vi "presets2 dialog.vi"(11 "Countries in":i32[](array[numeric])) -> (2 "Load?":bool, 3 "Countries out":i32[](array[numeric]))   [LabVIEW 2019]
uses:
  <vilib>/Utility/sysdir.llb/System Directory Type.ctl
  <vilib>/Utility/config.llb/Write Key (I32).vi
  <vilib>/Utility/config.llb/Read Key (I32).vi
  <vilib>/Utility/config.llb/NI_LVConfig.lvlib
panel:
  in  "Delete":bool
  in  "Load":bool
  in  "Save Button":bool
  in  "Cancel Button":bool
  in  "Presets":i32(listbox)
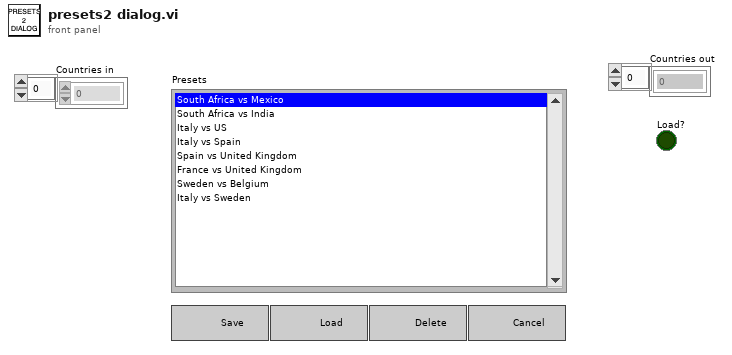
[diagram p1: front panel]
types:
  T1 = typedef "System Directory Type.ctl" = i32
  T2 = typedef "NI_LVConfig.lvlib/Config Data RefNum.ctl" = refnum<k1>
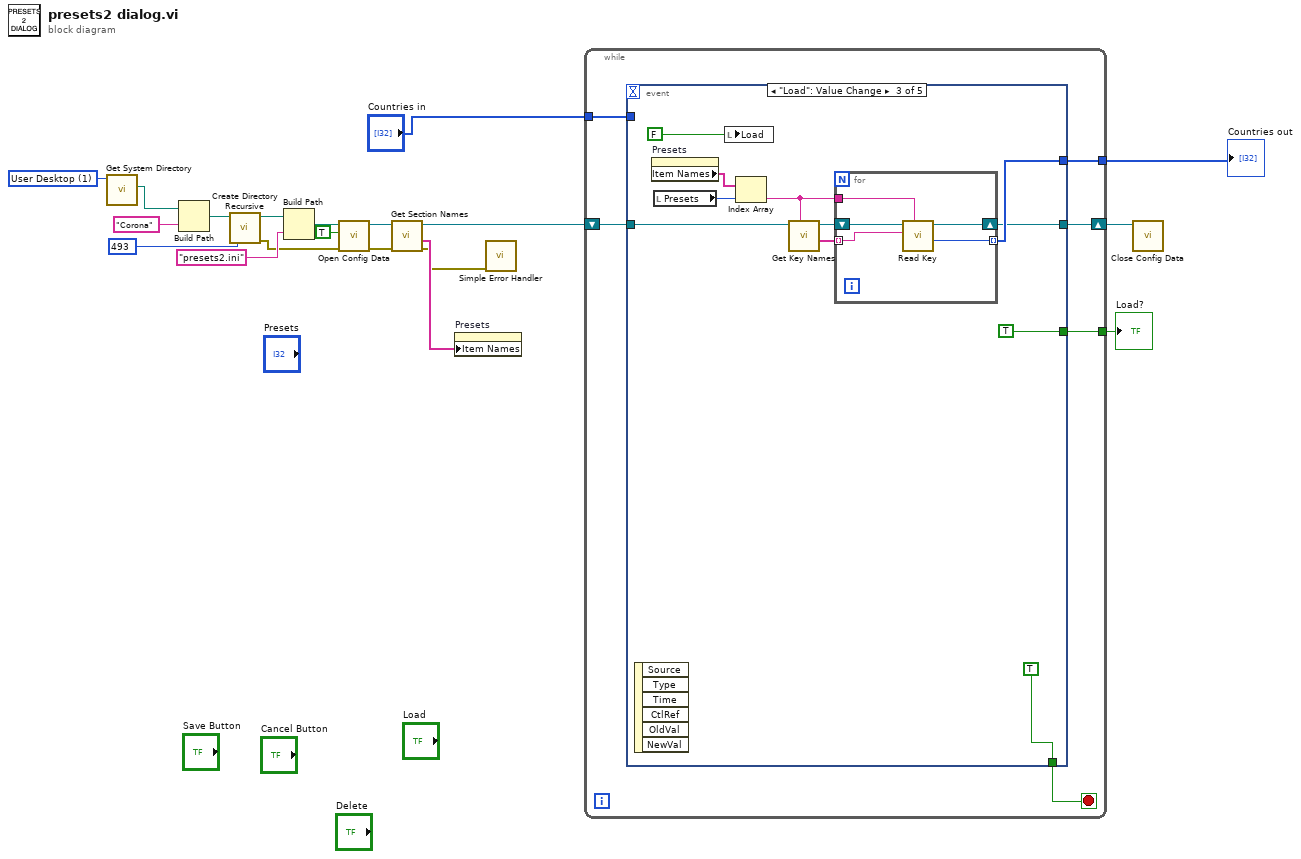
[diagram p0: block diagram]
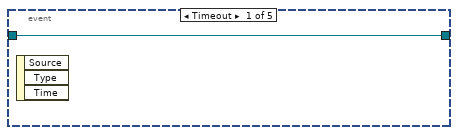
[diagram p2: hidden frame]
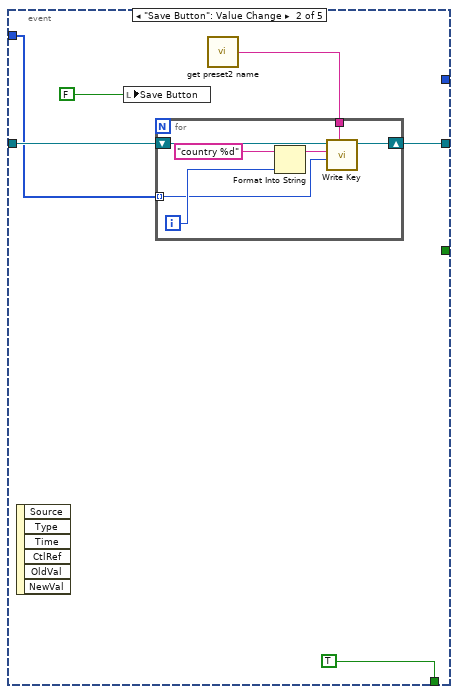
[diagram p3: hidden frame]
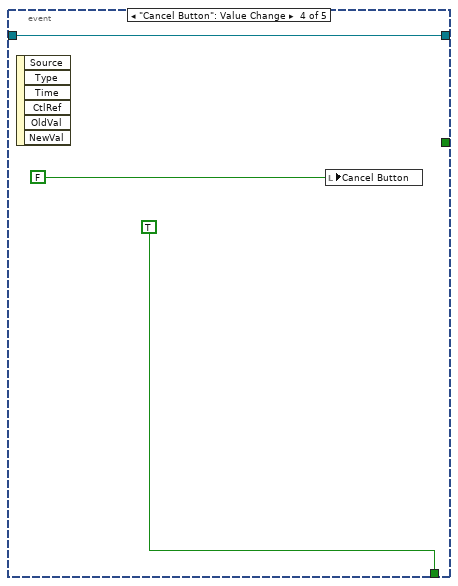
[diagram p4: hidden frame]
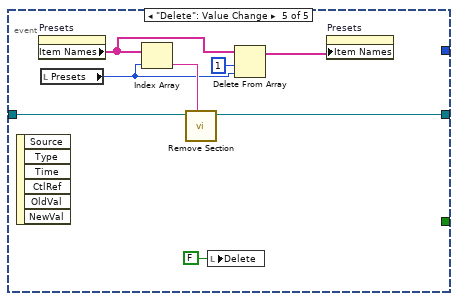
[diagram p5: hidden frame]
diagram:
  w19 = T1 1 items=["User Home"=0, "User Desktop"=1, "User Documents"=2, "User Application Data"=3, "User Preferences"=4, "User Temporary"=5, "Public Documents"=6, "Public Application Data"=7, "Public Preferences"=8, "Public Cache"=13, "System Core Libraries"=9, "System Installed Libraries"=10, "Application Files"=11, "Boot Volume Root"=12] ("system directory type")
  n1 = call <vilib>:"Get System Directory.vi"("system directory type"=w19) -> ("system directory"=w18:path)  [unwired: 10 in]
  n2 = Build Path(base path=w18, name or relative path="Corona") -> (appended path=w7:path)
  n3 = call <vilib>:"Create Directory Recursive.vi"("permissions"=i16 493, "directory"=w7) -> ("error out"=w5:errorcluster, "directory copy"=w6:path)  [unwired: 3 in, 1 out]
  n4 = Build Path(base path=w6, name or relative path="presets2.ini") -> (appended path=w15:path)
  n5 = call <vilib>:"Open Config Data.vi"("error in (no error)"=w5, "create file if necessary (T)"=TRUE, "configuration file path"=w15) -> ("error out"=w9:errorcluster, "refnum"=w13:T2)  [unwired: 6 in, 1 out]
  n6 = call <vilib>:"Get Section Names.vi"("error in (no error)"=w9, "refnum"=w13) -> ("error out"=w8:errorcluster, "section names"=w11:string[], "refnum out"=w12:T2)  [unwired: 7 in]
  n7 = property on="Presets" class="LstBox (strict)"("Item Names"=w11) -> ()  [unwired: 2 in, 2 out]
  n8 = call <vilib>:"Simple Error Handler.vi"("error in (no error)"=w8) -> ()  [unwired: 4 in, 5 out]
  n9 = while {
    shift-right: [w24] -> w10
    shift-left: w12 -> [w25]
    tunnel: "Countries in" -> [w22]
    tunnel: [w21] -> w2
    tunnel: [w20] -> w3
    stop <- w23 stop-if-true
    n10 = event shown="[2] \"Load\": Value Change" {
      selector: _ -> [_ _ _ _ _]
      dyn-events: _ -> [_ _ _ _ _]
      timeout: _ -> [_ _ _ _ _]
      tunnel: w25 -> [w26 w32 w45 w57 w66]
      tunnel: [w26 w27 w41 w57 w64] -> w24
      tunnel: [_ TRUE TRUE TRUE _] -> w23
      tunnel: w22 -> [_ w28 _ _ _]
      tunnel: [_ _ w42 _ _] -> w21
      tunnel: [_ _ TRUE _ _] -> w20
      event Timeout {
        n11 = event-data() -> ()  [unwired: 1 in, 3 out]
      }
      event "Save Button": Value Change {
        n12 = event-data() -> ()  [unwired: 1 in, 6 out]
        n13 = local write "Save Button"(FALSE ("Save Button")) -> ()
        n14 = call "get preset2 name.vi"() -> ("Preset name out"=w29:string)  [unwired: 1 in]
        n15 = for {
          tunnel: w29 -> [w37]
          tunnel: w28 -> [w34] mode=indexing
          shift-right: [w33] -> w27
          shift-left: w32 -> [w39]
          i -> [w35]
          n16 = Format Into String(initial string="country %d" ("key"), w35) -> (resulting string=w36:string)  [unwired: 2 in, 1 out]
          n17 = call-poly <vilib>:"Write Key.vi"("section"=w37, "value"=w34, "key"=w36, "refnum"=w39) -> ("refnum out"=w33:T2)  [unwired: 5 in, 2 out]
        }
      }
      event "Load": Value Change {
        n18 = event-data() -> ()  [unwired: 1 in, 6 out]
        n19 = property on="Presets" class="LstBox (strict)"() -> ("Item Names"=w48:string[])  [unwired: 2 in, 2 out]
        n20 = local read "Presets"() -> (w47:i32)
        n21 = local write "Load"(FALSE ("Save Button")) -> ()
        n22 = Index Array(array=w48, index=w47) -> (element=w40:string)
        n23 = call <vilib>:"Get Key Names.vi"("section"=w40, "refnum"=w45) -> ("key names"=w43:string[], "refnum out"=w44:T2)  [unwired: 6 in, 2 out]
        n24 = for {
          tunnel: w43 -> [w52] mode=indexing
          shift-right: [w54] -> w41
          shift-left: w44 -> [w55]
          tunnel: [w53] -> w42 mode=indexing
          tunnel: w40 -> [w51]
          n25 = call-poly <vilib>:"Read Key.vi"("section"=w51, "key"=w52, "refnum"=w55) -> ("value"=w53:i32, "refnum out"=w54:T2)  [unwired: 5 in, 2 out]
        }
      }
      event "Cancel Button": Value Change {
        n26 = event-data() -> ()  [unwired: 1 in, 6 out]
        n27 = local write "Cancel Button"(FALSE ("Cancel Button")) -> ()
      }
      event "Delete": Value Change {
        n28 = event-data() -> ()  [unwired: 1 in, 6 out]
        n29 = property on="Presets" class="LstBox (strict)"() -> ("Item Names"=w63:string[])  [unwired: 2 in, 2 out]
        n30 = local read "Presets"() -> (w61:i32)
        n31 = Index Array(array=w63, index=w61) -> (element=w65:string)
        n32 = call <vilib>:"Remove Section.vi"("section"=w65, "refnum"=w66) -> ("refnum out"=w64:T2)  [unwired: 7 in, 2 out]
        n33 = local write "Delete"(FALSE ("Delete")) -> ()
        n34 = Delete From Array(array=w63, length=1, index=w61) -> (array with subset deleted=w62:string[])  [unwired: 1 out]
        n35 = property on="Presets" class="LstBox (strict)"("Item Names"=w62) -> ()  [unwired: 2 in, 2 out]
      }
    }
  }
  "Load?" <- w3
  "Countries out" <- w2
  n36 = call <vilib>:"Close Config Data.vi"("refnum"=w10) -> ()  [unwired: 9 in, 2 out]
